vi "ZMC Check3File.vi"(7 "pFileSize":u32, 8 "error in (no error)":errorcluster caption="错误输入（无错误）", 9 "pbIfExist":string, 10 "pfilenameinControl":string, 11 "handle":u32) -> (0 "error out":errorcluster caption="错误输出", 1 "pbIfExist out":string, 2 "function return":i32, 3 "handle out":u32, 5 "pFileSize out":u32)   [LabVIEW 2015, in "zauxdll.lvlib"]
doc: "int32 __stdcall ZMC_Check3File(ZMC_HANDLE handle, const char* pfilenameinControl, uint8 *pbIfExist, uint32 *pFileSize);"
uses:
  zauxdll.lvlib
  zmotion.dll
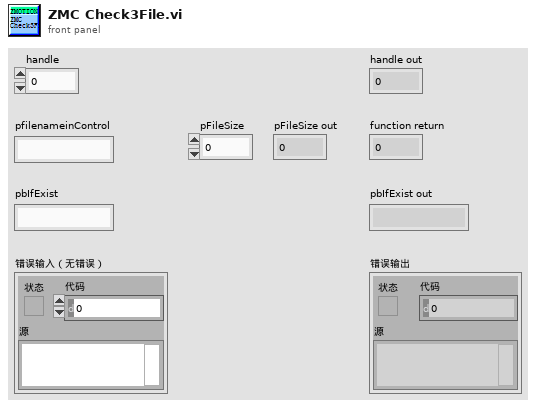
[diagram p1: front panel]
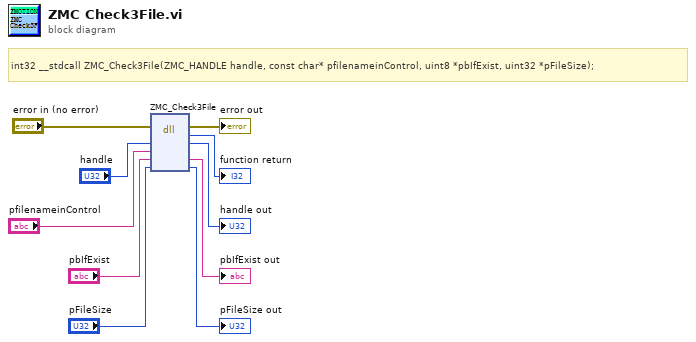
[diagram p0: block diagram]
diagram:
  # "int32 __stdcall ZMC_Check3File(ZMC_HANDLE handle, const char* pfilenameinControl, uint8 *pbIfExist, uint32 *pFileSize);"
  n1 = dll-call lib="C:/Users/VIC/Desktop/GOGORO_SA/system/LLB/zmotion/zaux/zmotion.*" fn="ZMC_Check3File"(error in="error in (no error)", "handle"="handle", "pfilenameinControl"="pfilenameinControl", "pbIfExist"="pbIfExist", "pFileSize"="pFileSize") -> (error out=→"error out":errorcluster, →"function return":i32, "handle"=→"handle out":u32, "pbIfExist"=→"pbIfExist out":string, "pFileSize"=→"pFileSize out":u32)  [unwired: 3 in, 1 out]
